vi "CSM - State Dashboard - DebugTool.vi"() -> ()   [LabVIEW 2014]
uses:
  _Support/Typedef/_CSM_GlobalLog_MSG.ctl
  _Support/Typedef/_CSM_GlobalLog_MSG_TYPE.ctl
  _Support/GlobalEvent/FGV-GlobalEventRef.vi
  <resource>/dialog/lvconfig.llb/LV Config Write Numeric (I32).vi
  <resource>/dialog/lvconfig.llb/LV Config Read Numeric (I32).vi
  _Support/jkism-tool-support.lvlib
  Communicable State Machine.lvlib
panel:
  in  "Clear JKISM":bool
  out "Dashboard":T1(array[cluster])
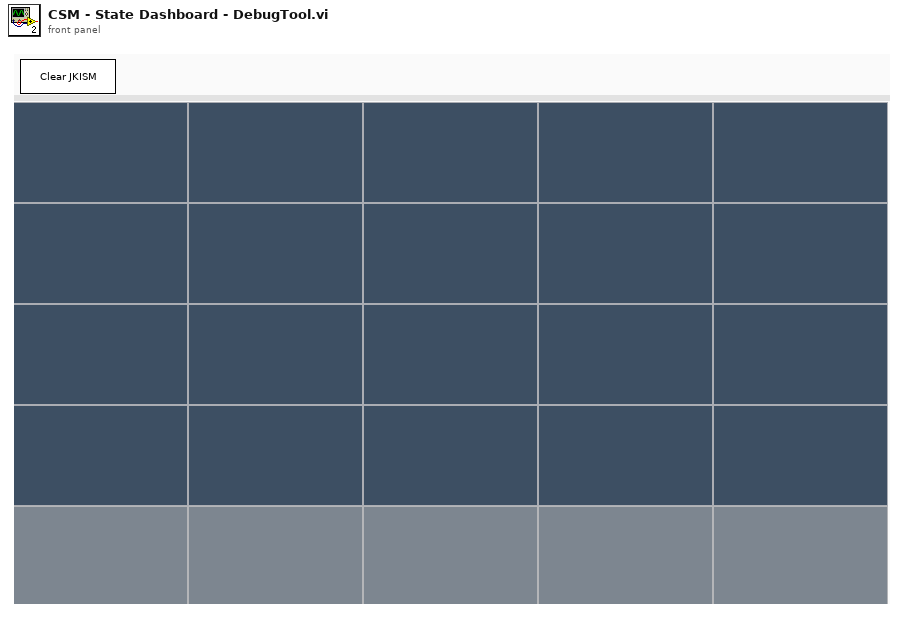
[diagram p1: front panel]
types:
  T1 = cluster{"Label":string, "Value":string, "String":string}[][]
  T2 = enum32{"Invalid", "Standard", "Closed", "Hidden", "Minimized", "Maximized"}
  T3 = enum32{"invalid app kind", "Development System", "Run Time System", "Student Edition", "Embedded LabVIEW", "Evaluation", "Custom"}
  T4 = typedef "Communicable State Machine.lvlib/_CSM_GlobalLog_MSG.ctl" = cluster{"Name(\"\" to use uuid)":string, "Current State":string, "Arguments":string, "Argument - State":string, "From Who":string, "Complete(T)/Start(F)":bool, "Type":T5}
  T5 = typedef "Communicable State Machine.lvlib/_CSM_GlobalLog_MSG_TYPE.ctl" = enum16{"User Log", "State Change", "Status", "Interrupt", "Register", "Unregister"}
  T6 = cluster{"Label":string, "Value":string, "String":string}
  T7 = typedef "JKI State Machine++.lvlib/_JKISM_GlobalLog_MSG_TYPE.ctl" = enum16{"User Log", "State Change", "Status", "Interrupt", "Register", "Unregister"}
  T8 = cluster{"Core":cluster{"Current VI Reference":refnum<vi>, "Close Panel on Exit?":bool}, "Global-DataTable":string[][], "NumCols":i16, "NumRows":i16, "JKISM Global Log Event":refnum<user-event>, "Log":T4}
  T9 = cluster{"Current VI Reference":refnum<vi>, "Close Panel on Exit?":bool}
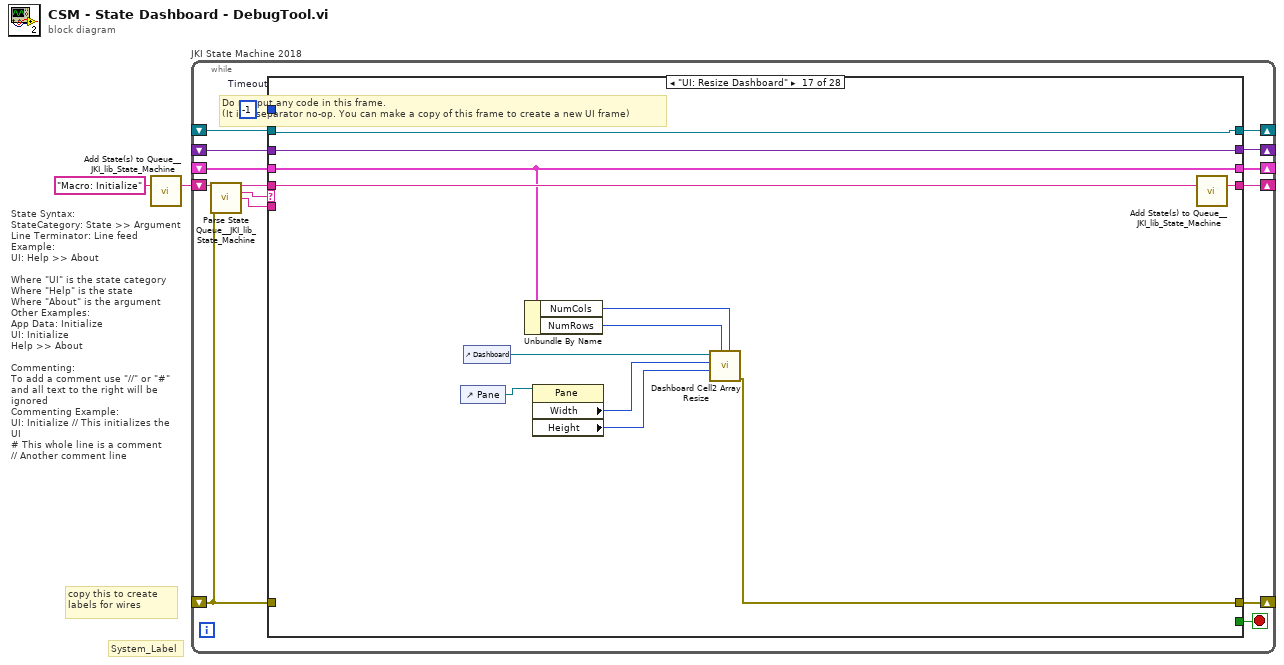
[diagram p0: block diagram]
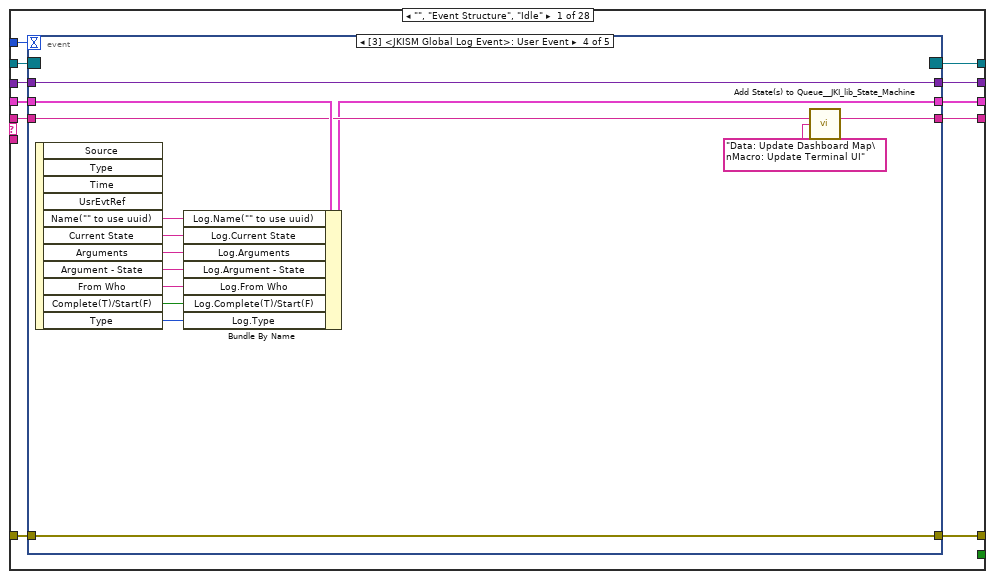
[diagram p2: hidden frame]
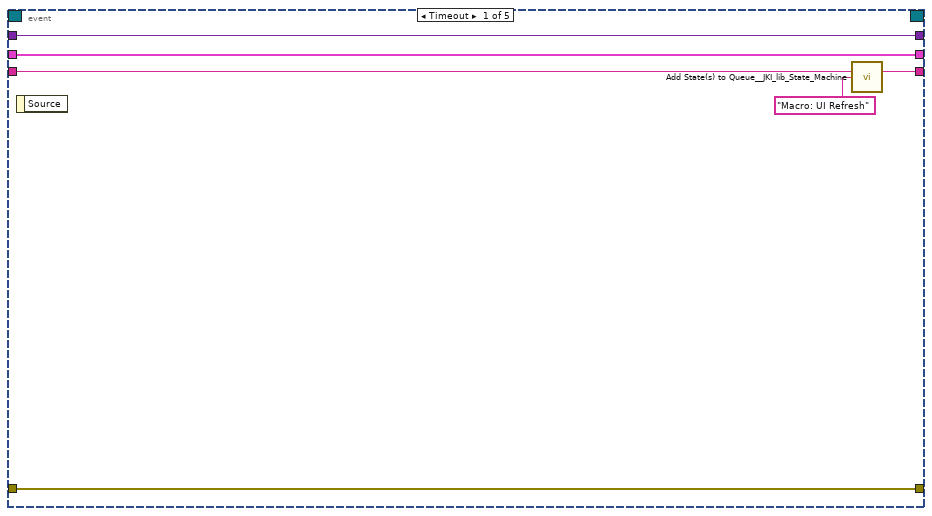
[diagram p3: hidden frame]
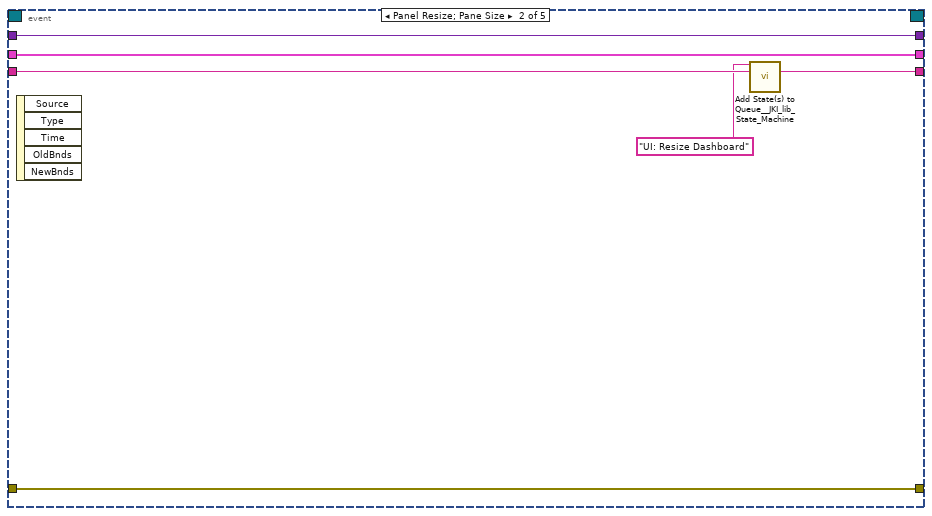
[diagram p4: hidden frame]
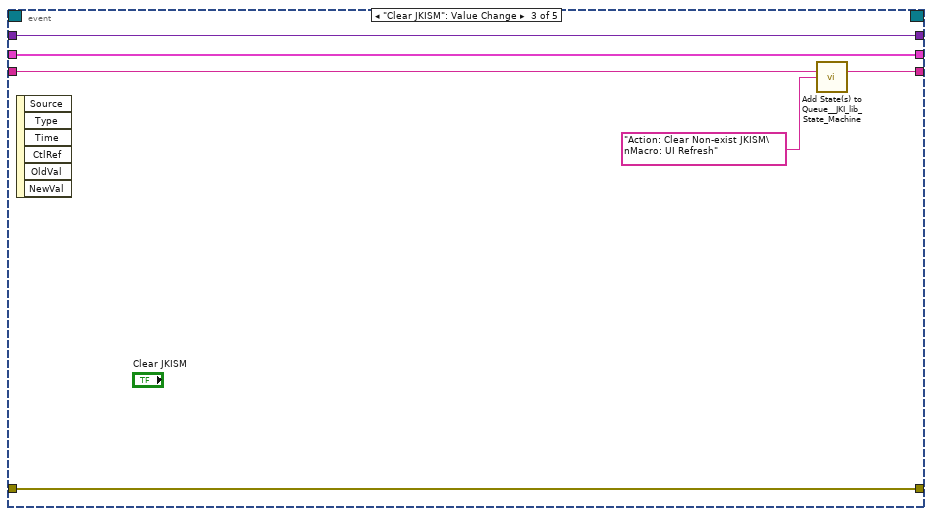
[diagram p5: hidden frame]
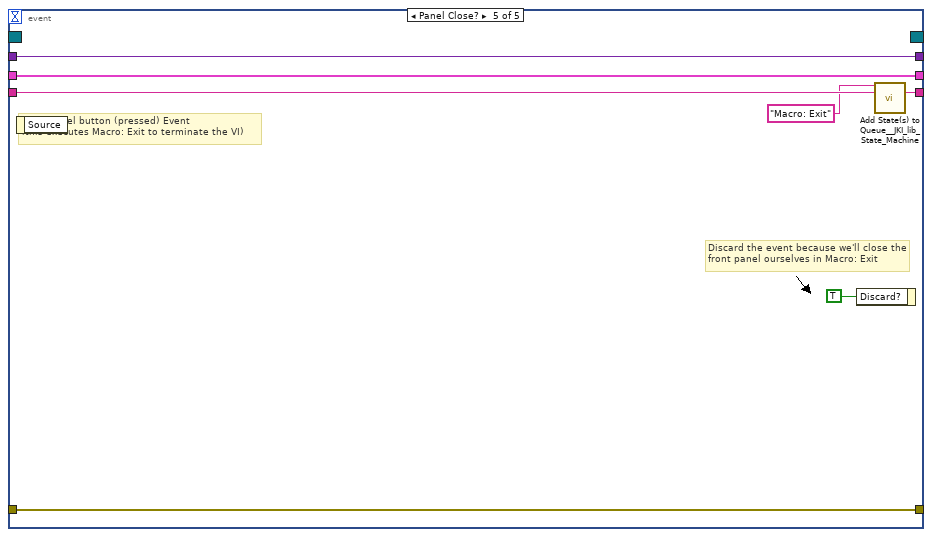
[diagram p6: hidden frame]
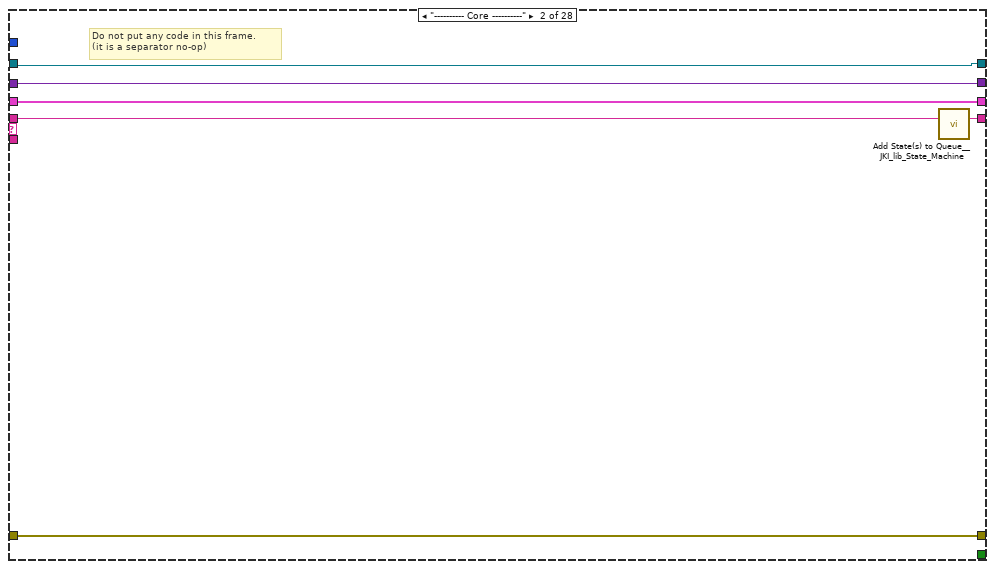
[diagram p7: hidden frame]
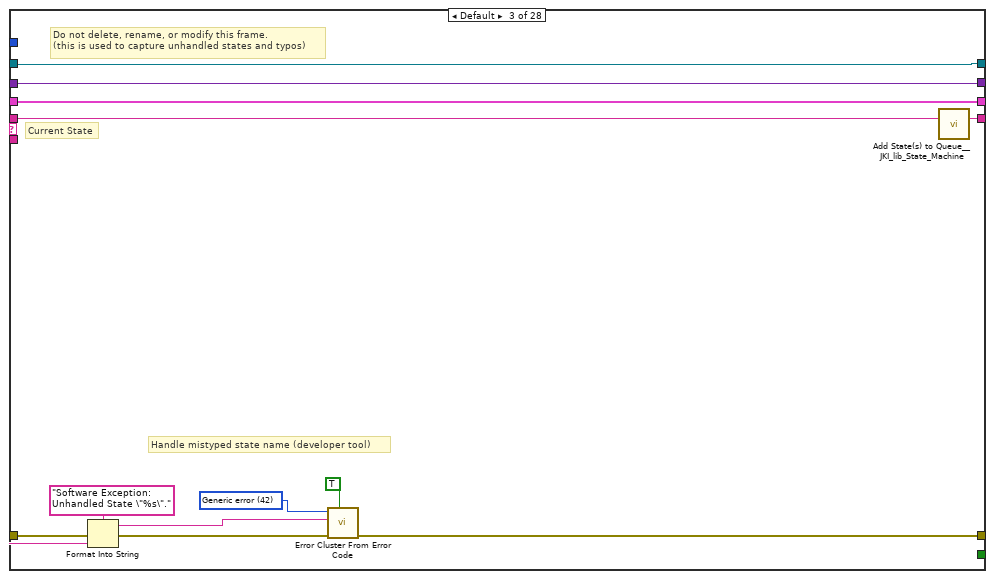
[diagram p8: hidden frame]
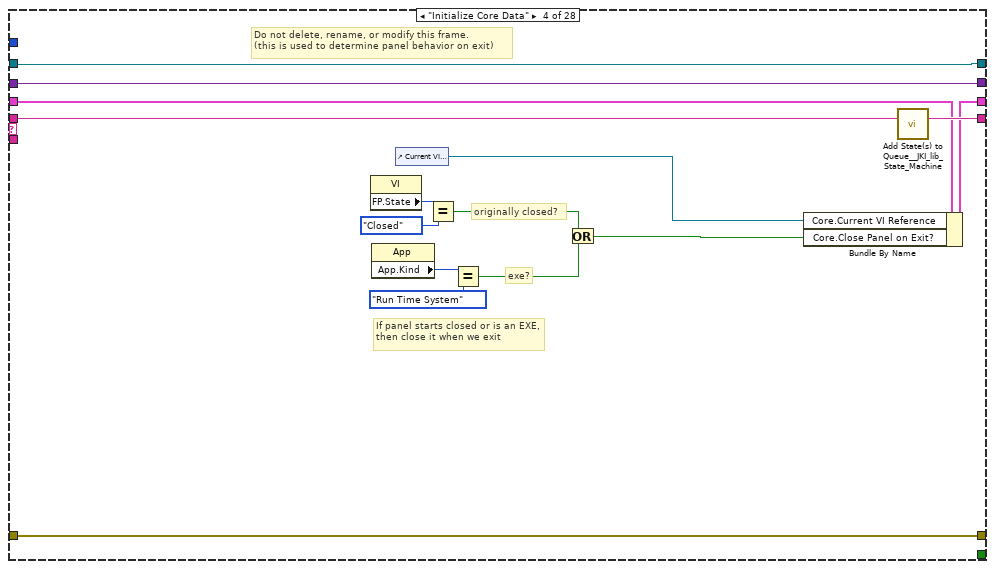
[diagram p9: hidden frame]
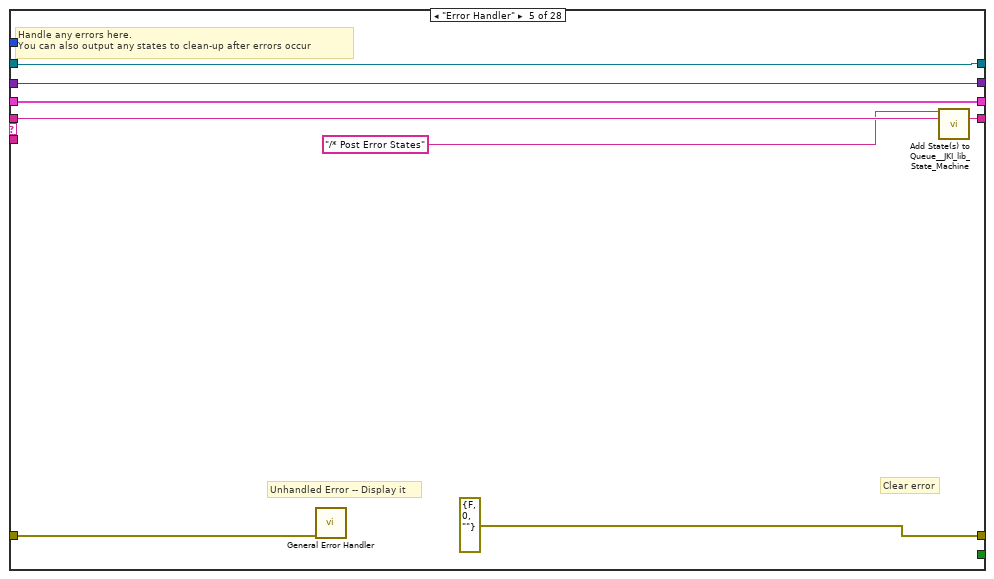
[diagram p10: hidden frame]
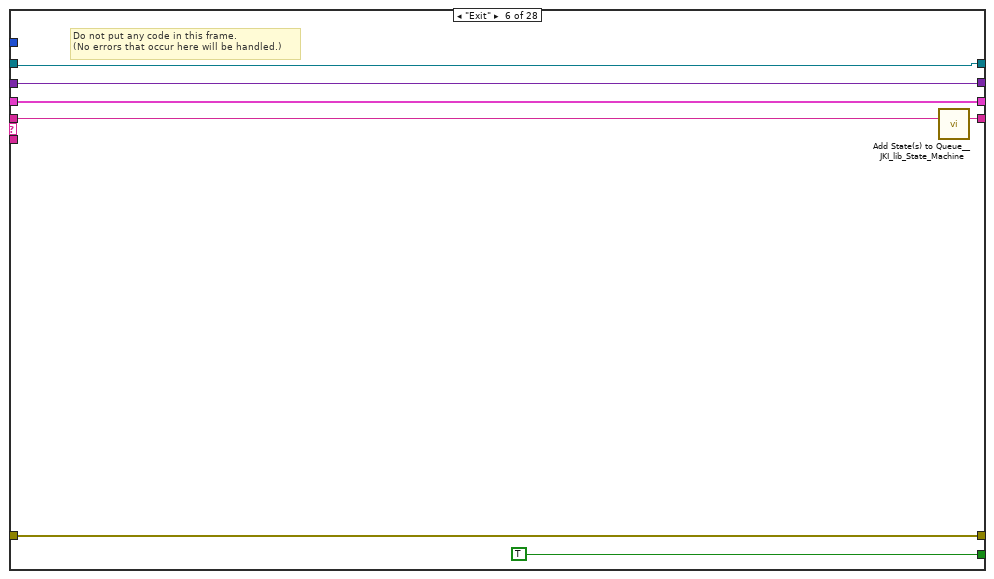
[diagram p11: hidden frame]
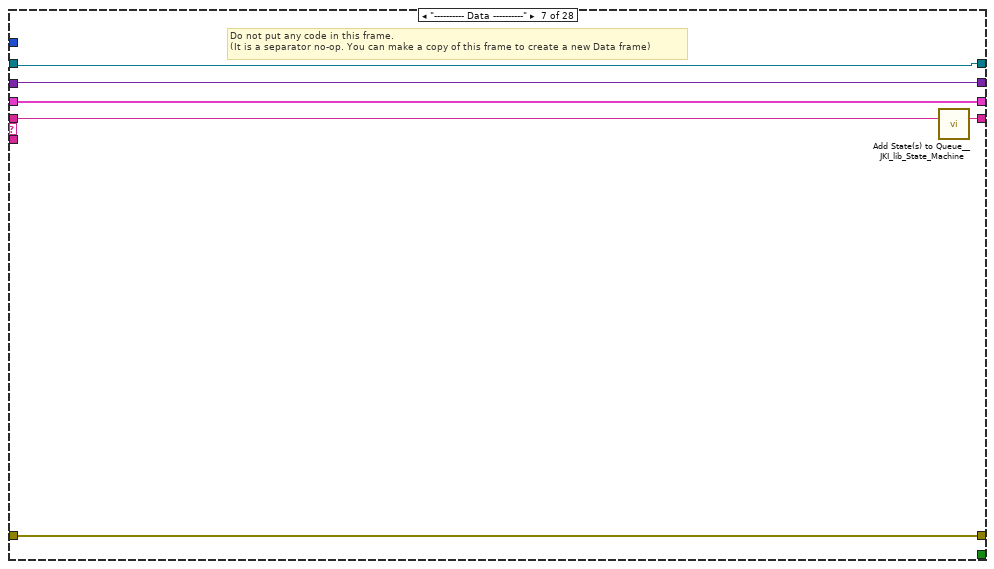
[diagram p12: hidden frame]
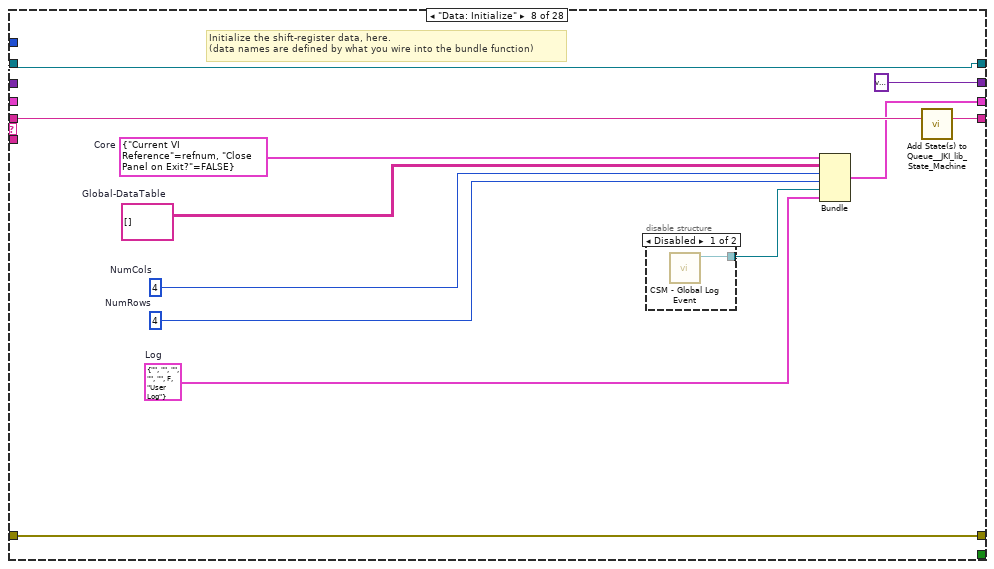
[diagram p13: hidden frame]
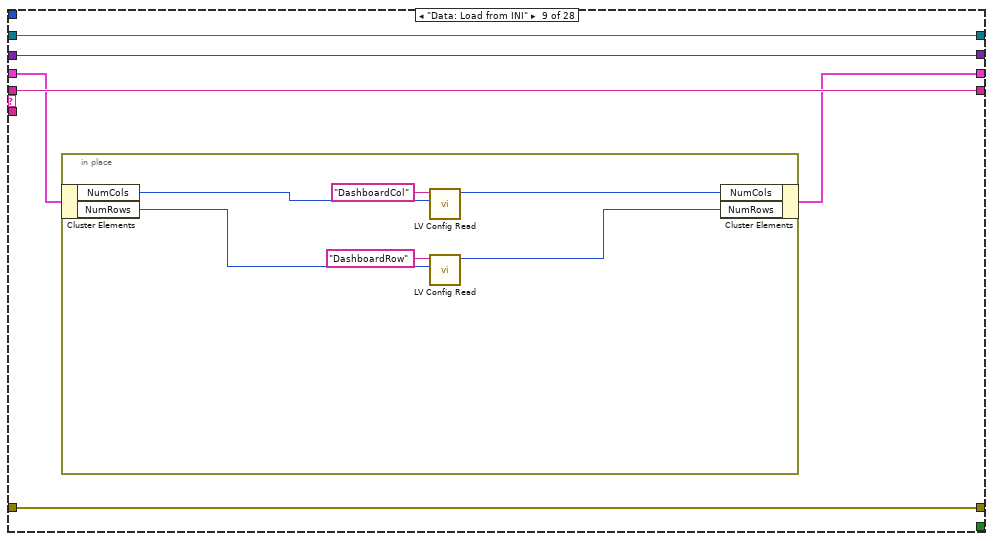
[diagram p15: hidden frame]
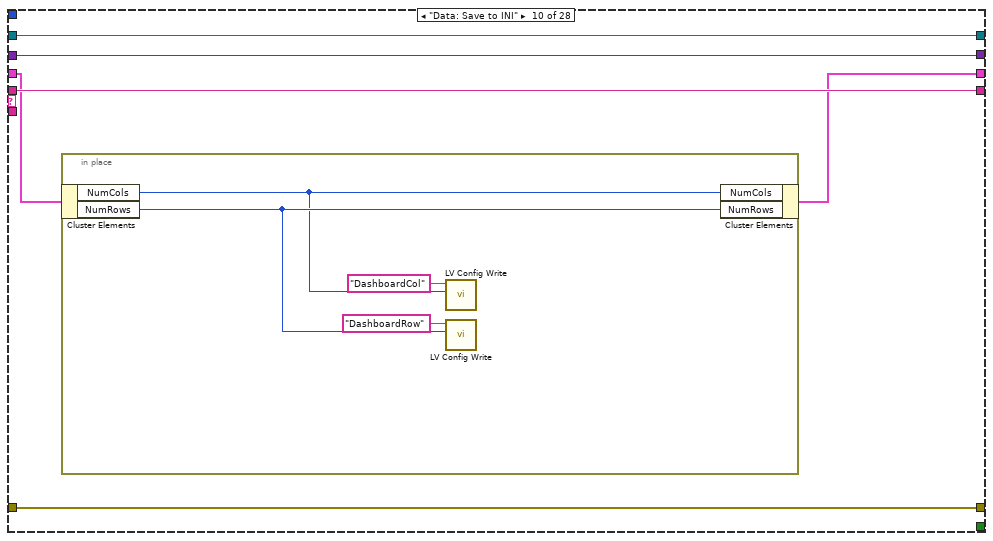
[diagram p16: hidden frame]
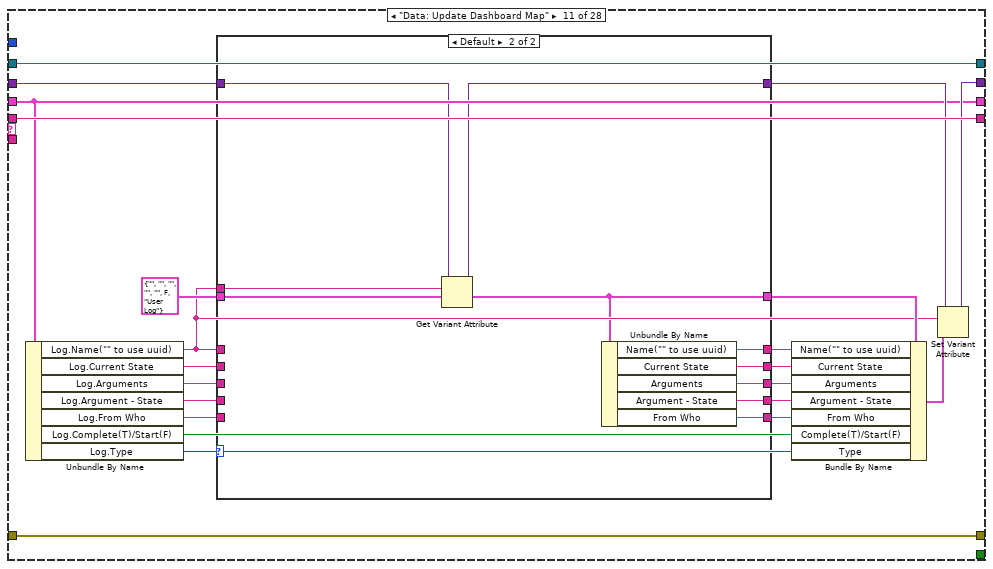
[diagram p17: hidden frame]
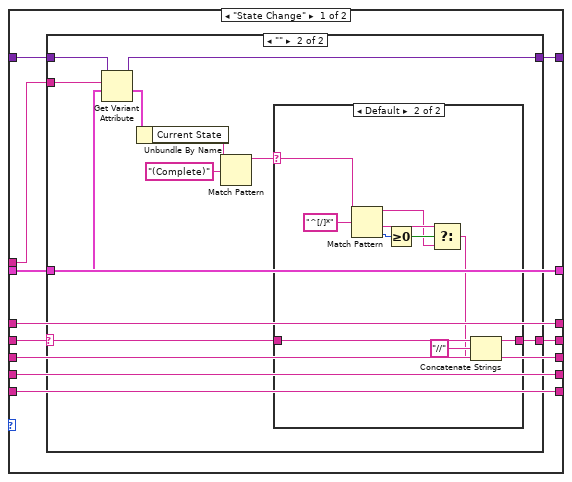
[diagram p18: hidden frame]
diagram:
  # "State Syntax:\nStateCategory: State >> Argument\nLine Terminator: Line feed\nExample:\nUI: Help >> About\n\nWhere \"UI\" is the state category\nWhere \"Help\" is the state\nWhere \"About\" is the argument\nOther Examples:\nApp Data: Initialize\nUI: Initialize\nHelp >> About\n\nCommenting:\nTo add a comment use \"//\" or \"#\" and all text to the right will be ignored\nCommenting Example:\nUI: Initialize // This initializes the UI\n# This whole line is a comment\n// Another comment line"
  # "copy this to create labels for wires"
  # "System_Label"
  n1 = call <vilib>:"Add State(s) to Queue__JKI_lib_State_Machine.vi"("State(s) in (\"\")"="Macro: Initialize") -> ("States Out"=w1:string)  [unwired: 14 in]
  n2 = while "JKI State Machine 2018" {
    shift-right: [w10] -> _
    shift-left: _ -> [w9]
    shift-right: [w13] -> _
    shift-left: _ -> [w7]
    shift-right: [w12] -> _
    shift-left: w1 -> [w14]
    shift-right: [w6] -> _
    shift-left: _ -> [w5]
    shift-right: [w4] -> _
    shift-left: _ -> [w3]
    stop <- w11 stop-if-true
    w8 = -1  # Timeout
    n3 = call <vilib>:"Parse State Queue__JKI_lib_State_Machine.vi"("State Queue"=w14, "Error In (no error)"=w7) -> ("Remaining States"=w16:string, "Current State"=w17:string, "Arguments"=w15:string)  [unwired: 11 in]
    n4 = case shown="\"UI: Resize Dashboard\"" w17 {
      selector: w17 -> [_ _ w76 _ _ _ _ _ _ _ _ _ _ _ _ _ _ _ _ _ _ _ _ _ _ _ _ _]
      tunnel: w16 -> [w28 w73 w80 w101 w109 w116 w122 w134 w140 w152 w178 w231 w237 w246 w258 w271 w348 w363 w373 w381 w389 w396 w403 w411 w418 w431 w435 w446]
      tunnel: w15 -> [_ _ _ _ _ _ _ _ _ _ _ _ _ _ w253 w265 _ _ _ _ _ _ _ _ _ _ _ _]
      tunnel: w9 -> [w26 w70 w78 w94 w106 w114 w119 _ w139 w151 w165 w226 w234 w242 w256 w267 w344 w360 w372 w380 w385 w393 w400 w406 w415 w428 w434 w445]
      tunnel: [w25 w71 w82 w98 errorcluster {"status"=FALSE, "code"=0, "source"=""} ("error out") w113 w120 w130 w141 w153 w179 w225 w235 w244 w254 w268 w345 w361 w374 w382 w390 w394 w401 w409 w416 w429 w436 w447] -> w13
      tunnel: w7 -> [w24 w71 w81 w98 w105 w113 w120 w130 w141 w153 w179 w228 w235 w244 w255 w269 _ w361 w374 w382 w390 w394 w401 w409 w416 w429 w436 w447]
      tunnel: [w27 w72 w79 w100 w108 w115 w121 w133 w140 w152 w178 w230 w236 w245 w257 w270 w347 w362 w373 w381 w389 w395 w402 w410 w417 w430 w435 w446] -> w12
      tunnel: [_ _ _ _ _ TRUE _ _ _ _ _ _ _ _ _ _ _ _ _ _ _ _ _ _ _ _ _ _] -> w11
      tunnel: [w23 w70 w78 w99 w106 w114 w119 w132 w138 w150 w165 w226 w234 w242 w256 w267 w344 w360 w372 w376 w385 w393 w400 w406 w415 w428 w434 w445] -> w10
      tunnel: w8 -> [w22 _ _ _ _ _ _ _ _ _ _ _ _ _ _ _ _ _ _ _ _ _ _ _ _ _ _ _]
      tunnel: [w20 w69 w75 w88 w103 w111 w118 variant w137 w149 w166 w224 w233 w239 w252 w264 w341 w355 w371 w379 w388 w392 w398 w405 w413 w421 w433 w441] -> w6
      tunnel: w5 -> [w21 w69 w75 w88 w103 w111 w118 _ w137 w149 w167 w224 w233 w239 w252 w264 w341 w354 w371 w379 w388 w392 w398 w405 w413 w421 w433 w443]
      tunnel: [w18 w68 w74 w87 w102 w110 w117 w125 w136 w148 w177 w223 w232 w238 w251 w263 w340 w351 w370 w377 w387 w391 w397 w404 w412 w420 w432 w444] -> w4
      tunnel: w3 -> [w19 w68 w74 w87 w102 w110 w117 w125 w136 w148 w177 w223 w232 w238 w251 w263 w340 w351 w370 _ w387 w391 w397 w404 w412 w420 w432 w444]
      frame "", "Event Structure", "Idle" {
        n5 = event shown="[3] <JKISM Global Log Event>: User Event" {
          selector: w19 -> [_ _ _ _ _]
          dyn-events: [_ _ _ _ _] -> w18
          timeout: w22 -> [_ _ _ _ _]
          tunnel: w28 -> [w34 w37 w43 w55 w67]
          tunnel: [w33 w38 w42 w59 w66] -> w27
          tunnel: w26 -> [w31 w39 w45 w56 w65]
          tunnel: [w32 w40 w46 w60 w62] -> w25
          tunnel: w24 -> [w32 w40 w46 w60 w62]
          tunnel: [w31 w39 w45 w54 w65] -> w23
          tunnel: w21 -> [w29 w35 w44 w57 w61]
          tunnel: [w29 w35 w44 w57 w61] -> w20
          event Timeout {
            n6 = event-data() -> ()  [unwired: 1 in, 1 out]
            n7 = call <vilib>:"Add State(s) to Queue__JKI_lib_State_Machine.vi"("State(s) in (\"\")"=w34, "State(s) at Back (\"\")"="Macro: UI Refresh" ("State(s) in Front (\"\")")) -> ("States Out"=w33:string)  [unwired: 13 in]
          }
          event Panel Resize; Pane Size {
            n8 = event-data() -> ()  [unwired: 1 in, 5 out]
            n9 = call <vilib>:"Add State(s) to Queue__JKI_lib_State_Machine.vi"("State(s) in Front (\"\")"="UI: Resize Dashboard" ("State(s) in Front (\"\")"), "State(s) in (\"\")"=w37) -> ("States Out"=w38:string)  [unwired: 13 in]
          }
          event "Clear JKISM": Value Change {
            n10 = event-data() -> ()  [unwired: 1 in, 6 out]
            n11 = call <vilib>:"Add State(s) to Queue__JKI_lib_State_Machine.vi"("State(s) in (\"\")"=w43, "State(s) at Back (\"\")"="Action: Clear Non-exist JKISM\nMacro: UI Refresh" ("State(s) at Back (\"\")")) -> ("States Out"=w42:string)  [unwired: 13 in]
          }
          event User Event {
            n12 = event-data() -> ("Name(\"\" to use uuid)"=w48:string, "Current State"=w49:string, "Arguments"=w50:string, "Argument - State"=w51:string, "From Who"=w52:string, "Complete(T)/Start(F)"=w53:bool, "Type"=w47:T7)  [unwired: 1 in, 4 out]
            n13 = Bundle By Name(cluster=w56, "Log.Name(\"\" to use uuid)"=w48, "Log.Current State"=w49, "Log.Arguments"=w50, "Log.Argument - State"=w51, "Log.From Who"=w52, "Log.Complete(T)/Start(F)"=w53, "Log.Type"=w47) -> (w54:T8)
            n14 = call <vilib>:"Add State(s) to Queue__JKI_lib_State_Machine.vi"("State(s) in (\"\")"=w55, "State(s) at Back (\"\")"="Data: Update Dashboard Map\nMacro: Update Terminal UI" ("State(s) at Back (\"\")")) -> ("States Out"=w59:string)  [unwired: 13 in]
          }
          event Panel Close? {
            # "Discard the event because we'll close the front panel ourselves in Macro: Exit"
            # "Close Panel button (pressed) Event\n(this executes Macro: Exit to terminate the VI)"
            n15 = event-data() -> ()  [unwired: 1 in, 1 out]
            n16 = event-data("Discard?"=TRUE) -> ()  [unwired: 1 in, 1 out]
            n17 = call <vilib>:"Add State(s) to Queue__JKI_lib_State_Machine.vi"("State(s) in Front (\"\")"="Macro: Exit", "State(s) in (\"\")"=w67) -> ("States Out"=w66:string)  [unwired: 13 in]
          }
        }
      }
      frame "---------- Core ----------" {
        # "Do not put any code in this frame.\n(it is a separator no-op)"
        n18 = call <vilib>:"Add State(s) to Queue__JKI_lib_State_Machine.vi"("State(s) in (\"\")"=w73) -> ("States Out"=w72:string)  [unwired: 14 in]
      }
      frame Default {
        w85 = 42 items=["No error", "Argument error", "Memory is full", "Out of zone", "End of file", "File already open", "Generic file I/O error", "File not found", "File permission error", "Disk is full", "Duplicate path", "Too many files open", "System feature not enabled", "Resource file not found", "Cannot add resource", "Resource not found", "Image not found", "Image memory error", "Pen does not exist", "Config type invalid", "Config token not found", "Config parse error", "Config memory error", "Bad external code format", "Bad external code offset", "External code not present", "Null window", "Destroy window error", "Null menu", "Print aborted", "Bad print record", "Print driver error", "Windows error during printing", "Memory error during printing", "Print dialog error", "Generic print error", "Invalid device refnum", "Device not found", "Device parameter error", "Device unit error", "Cannot open device", "Device call aborted", "Generic error", "Cancelled by user", "Object ID too low", "Object ID too high", "Object not in heap", "Unknown heap", "Unknown object (invalid DefProc)", "Unknown object (DefProc not in table)", "Message out of range", "Invalid (null) method", "Unknown message", "Manager call not supported", "Bad address", "Network operation in progress", "Network operation timed out", "Connection is busy", "Network attribute not supported", "Network error", "Address in use", "System out of memory", "Connection aborted", "Connection refused", "Not connected", "Already connected", "Connection closed", "Initialization error (interapplication manager)", "Bad occurrence", "Wait on unbound occurrence handler", "Occurrence queue overflow", "Datalog type conflict", "Unused", "Unrecognized type (interapplication manager)", "Memory corrupt", "Failed to make temporary DLL", "Old CIN version", "Drag socket not found", "Failed to load drop-object", "Failed to register OLE object", "Failed to release OLE object", "Format specifier type mismatch", "Unknown format specifier", "Too few format specifiers", "Too many format specifiers", "Scan failed", "Newer CIN version", "Error converting to variant", "Runtime menu error", "Password tampered", "Variant attribute not found", "Incompatible variant data type", "Event data is not available", "Event Store is not present", "Occurrence is not found", "Event Queue is not created", "Event info is not available", "Refnum passed is NULL", "Error retrieving Class GUID", "Error retrieving CoClass GUID", "Error retrieving TypeLib GUID.", "Bad built application magic bytes.", "Specific driver is different from the specific driver associated with the Logical Name.", "There is no session opened to the class driver.", "Max Error", "MAX - Error with config objects", "MAX - Error loading configuration", "MAX - Group not supported"]
        # "Current State"
        # "Do not delete, rename, or modify this frame.\n(this is used to capture unhandled states and typos)"
        # "Handle mistyped state name (developer tool)"
        n19 = Format Into String(format string="Software Exception: Unhandled State \"%s\"." ("message"), error in=w81, w76) -> (resulting string=w84:string, error out=w83:errorcluster)  [unwired: 1 in]
        n20 = call <vilib>:"Error Cluster From Error Code.vi"("show call chain? (False)"=TRUE, "error in (no error)"=w83, "error message (\"\")"=w84, "error code (0)"=w85) -> ("error out"=w82:errorcluster)  [unwired: 5 in]
        n21 = call <vilib>:"Add State(s) to Queue__JKI_lib_State_Machine.vi"("State(s) in (\"\")"=w80) -> ("States Out"=w79:string)  [unwired: 14 in]
      }
      frame "Initialize Core Data" {
        # "Do not delete, rename, or modify this frame.\n(this is used to determine panel behavior on exit)"
        # "originally closed?"
        # "exe?"
        # "If panel starts closed or is an EXE, then close it when we exit"
        n22 = property class="VI"() -> ("FP.State"=w91:T2)  [unwired: 2 in, 2 out]
        n23 = property class="App"() -> ("App.Kind"=w97:T3)  [unwired: 2 in, 2 out]
        n24 = control-ref of="Current VI Reference"() -> (w92:refnum<vi>)
        n25 = Equal?(x=w91, y=T2."Closed" ("Front Panel Window:State")) -> (x = y?=w89:bool)
        n26 = Equal?(x=w97, y=T3."Run Time System" ("Application:Kind")) -> (x = y?=w95:bool)
        n27 = Or(x=w89, y=w95) -> (x .or. y?=w93:bool)
        n28 = Bundle By Name(cluster=w94, "Core.Current VI Reference"=w92, "Core.Close Panel on Exit?"=w93) -> (w99:T8)
        n29 = call <vilib>:"Add State(s) to Queue__JKI_lib_State_Machine.vi"("State(s) in (\"\")"=w101) -> ("States Out"=w100:string)  [unwired: 14 in]
      }
      frame "Error Handler" {
        # "Unhandled Error -- Display it"
        # "Handle any errors here.\nYou can also output any states to clean-up after errors occur"
        # "Clear error"
        n30 = call <vilib>:"General Error Handler.vi"("error in (no error)"=w105) -> ()  [unwired: 10 in, 5 out]
        n31 = call <vilib>:"Add State(s) to Queue__JKI_lib_State_Machine.vi"("State(s) in Front (\"\")"="/* Post Error States", "State(s) in (\"\")"=w109) -> ("States Out"=w108:string)  [unwired: 13 in]
      }
      frame "Exit" {
        # "Do not put any code in this frame.\n(No errors that occur here will be handled.)"
        n32 = call <vilib>:"Add State(s) to Queue__JKI_lib_State_Machine.vi"("State(s) in (\"\")"=w116) -> ("States Out"=w115:string)  [unwired: 14 in]
      }
      frame "---------- Data ----------" {
        # "Do not put any code in this frame.\n(It is a separator no-op. You can make a copy of this frame to create a new Data frame)"
        n33 = call <vilib>:"Add State(s) to Queue__JKI_lib_State_Machine.vi"("State(s) in (\"\")"=w122) -> ("States Out"=w121:string)  [unwired: 14 in]
      }
      frame "Data: Initialize" {
        w123 = T4 {"Name(\"\" to use uuid)"="", "Current State"="", "Arguments"="", "Argument - State"="", "From Who"="", "Complete(T)/Start(F)"=FALSE, "Type"=enum."User Log"}  # Log
        w128 = i16 4  # NumCols
        w127 = i16 4  # NumRows
        w129 = string[][] []  # Global-DataTable
        w131 = T9 {"Current VI Reference"=refnum, "Close Panel on Exit?"=FALSE}  # Core
        # "Initialize the shift-register data, here.\n(data names are defined by what you wire into the bundle function)"
        n34 = disable-structure shown="Disabled" {
          disable-tunnel: [w135 _] -> w124
          frame Disabled {
            n35 = call "CSM - Global Log Event.vi"() -> ("JKISM Global Log Event"=w135:refnum<user-event>)  [unwired: 10 in, 1 out]
          }
          frame Enabled {
          }
        }
        n36 = Bundle("Core"=w131, "Global-DataTable"=w129, "NumCols"=w128, "NumRows"=w127, "JKISM Global Log Event"=w124, "Log"=w123) -> (w132:T8)  [unwired: 1 in]
        n37 = call <vilib>:"Add State(s) to Queue__JKI_lib_State_Machine.vi"("State(s) in (\"\")"=w134) -> ("States Out"=w133:string)  [unwired: 14 in]
      }
      frame "Data: Load from INI" {
        n38 = in-place {
          n39 = in-place-cluster #1(w139) -> ("NumCols"=w143:i16, "NumRows"=w146:i16)
          n40 = call-poly <resource>:"LV Config Read.vi"("default value"=w143, "key"="DashboardCol") -> ("value"=w142:i32)  [unwired: 3 in, 2 out]
          n41 = call-poly <resource>:"LV Config Read.vi"("default value"=w146, "key"="DashboardRow") -> ("value"=w145:i32)  [unwired: 3 in, 2 out]
          n42 = in-place-cluster #1("NumCols"=w142, "NumRows"=w145) -> (w138:T8)
        }
      }
      frame "Data: Save to INI" {
        n43 = in-place {
          n44 = in-place-cluster #2(w151) -> ("NumCols"=w154:i16, "NumRows"=w155:i16)
          n45 = call-poly <resource>:"LV Config Write.vi"("value"=w154, "key"="DashboardCol") -> ()  [unwired: 5 in, 1 out]
          n46 = call-poly <resource>:"LV Config Write.vi"("value"=w155, "key"="DashboardRow") -> ()  [unwired: 5 in, 1 out]
          n47 = in-place-cluster #2("NumCols"=w154, "NumRows"=w155) -> (w150:T8)
        }
      }
      frame "Data: Update Dashboard Map" {
        n48 = Unbundle By Name(w165) -> ("Log.Name(\"\" to use uuid)"=w160:string, "Log.Current State"=w164:string, "Log.Arguments"=w163:string, "Log.Argument - State"=w162:string, "Log.From Who"=w161:string, "Log.Complete(T)/Start(F)"=w158:bool, "Log.Type"=w159:T5)
        n49 = case shown="Default" w159 {
          tunnel: w167 -> [w185 w222]
          tunnel: [w184 w221] -> w175
          tunnel: T4 {"Name(\"\" to use uuid)"="", "Current State"="", "Arguments"="", "Argument - State"="", "From Who"="", "Complete(T)/Start(F)"=FALSE, "Type"=enum."User Log"} ("Cross JKI State Machine Data") -> [w182 w220]
          tunnel: w160 -> [w183 w219]
          tunnel: w161 -> [w189 _]
          tunnel: [w189 w218] -> w173
          tunnel: w162 -> [w188 _]
          tunnel: [w188 w217] -> w172
          tunnel: w163 -> [w187 _]
          tunnel: [w187 w216] -> w171
          tunnel: w164 -> [w181 _]
          tunnel: [w180 w213] -> w170
          tunnel: w160 -> [w186 _]
          tunnel: [w186 w214] -> w169
          tunnel: [w182 w215] -> w168
          frame "State Change" {
            n50 = case shown="\"\"" w181 {
              selector: w181 -> [w190 w193]
              tunnel: w185 -> [w191 w201]
              tunnel: [w191 w200] -> w184
              tunnel: w183 -> [_ w199]
              tunnel: w182 -> [_ w197]
              tunnel: [w190 w192] -> w180
              frame Default {
              }
              frame "" {
                n51 = Get Variant Attribute(Variant=w201, name=w199, default value (empty Variant)=w197) -> (duplicate Variant=w200:variant, value=w198:T4)  [unwired: 1 in, 2 out]
                n52 = Unbundle By Name(w198) -> ("Current State"=w196:string)
                n53 = Match Pattern(string=w196, regular expression="(Complete)") -> (before substring=w194:string)  [unwired: 1 in, 3 out]
                n54 = case shown="Default" w194 {
                  selector: w194 -> [_ w208]
                  tunnel: w193 -> [w202 w212]
                  tunnel: [w202 w211] -> w192
                  frame "" {
                  }
                  frame Default {
                    n55 = Match Pattern(string=w208, regular expression="^[/]*") -> (before substring=w203:string, after substring=w205:string, offset past match=w207:i32)  [unwired: 1 in, 1 out]
                    n56 = Greater Or Equal To 0?(x=w207) -> (x >= 0?=w206:bool)
                    n57 = Select(t=w205, s=w206, f=w203) -> (s? t:f=w204:string)
                    n58 = Concatenate Strings(w212, "//" ("string"), w204) -> (w211:string)
                  }
                }
              }
            }
          }
          frame Default {
            n59 = Get Variant Attribute(Variant=w222, name=w219, default value (empty Variant)=w220) -> (duplicate Variant=w221:variant, value=w215:T4)  [unwired: 1 in, 2 out]
            n60 = Unbundle By Name(w215) -> ("Name(\"\" to use uuid)"=w214:string, "Current State"=w213:string, "Arguments"=w216:string, "Argument - State"=w217:string, "From Who"=w218:string)
          }
        }
        n61 = Bundle By Name(cluster=w168, "Name(\"\" to use uuid)"=w169, "Current State"=w170, "Arguments"=w171, "Argument - State"=w172, "From Who"=w173, "Complete(T)/Start(F)"=w158, "Type"=w159) -> (w176:T4)
        n62 = Set Variant Attribute(Variant=w175, name=w160, value=w176) -> (Variant out=w166:variant)  [unwired: 1 in, 2 out]
      }
      frame "Data: Cleanup" {
        # "Cleanup any data and references, here.\n(this is called automatically, by the Macro: Exit)"
        n63 = Unbundle By Name(w226) -> ("Core.Current VI Reference"=w229:refnum<vi>)
        n64 = Close Reference(reference=w229, error in (no error)=w228) -> (error out=w227:errorcluster)
        n65 = Merge Errors(w227) -> (w225:errorcluster)
        n66 = call <vilib>:"Add State(s) to Queue__JKI_lib_State_Machine.vi"("State(s) in (\"\")"=w231) -> ("States Out"=w230:string)  [unwired: 14 in]
      }
      frame "---------- UI ----------" {
        # "Do not put any code in this frame.\n(It is a separator no-op. You can make a copy of this frame to create a new UI frame)"
        n67 = call <vilib>:"Add State(s) to Queue__JKI_lib_State_Machine.vi"("State(s) in (\"\")"=w237) -> ("States Out"=w236:string)  [unwired: 14 in]
      }
      frame "UI: Initialize" {
        # "Initialize the User Interface, here.\n(this is called automatically, by the Macro: Init)"
        n68 = invoke class="VI" method="Default Vals.Reinit All"() -> (error out=w243:errorcluster)  [unwired: 3 in, 2 out]
        n69 = Unbundle By Name(w242) -> ("NumRows"=w241:i16, "NumCols"=w240:i16)
        n70 = flat-sequence {
          tunnel: w243 -> [_]
          tunnel: w241 -> [w248]
          tunnel: w240 -> [w247]
          frame #0 {
            n71 = Initialize Array(T6 {"Label"="", "Value"="", "String"=""} ("Dashboard"), w248, w247) -> (w249:T1)
            n72 = local write "Dashboard"(w249) -> ()
          }
        }
        n73 = call <vilib>:"Add State(s) to Queue__JKI_lib_State_Machine.vi"("State(s) in (\"\")"=w246) -> ("States Out"=w245:string)  [unwired: 14 in]
      }
      frame "UI: Cursor Set" {
        # "Argument"
        # "Set and Unset Cursor Busy.\n(Usage: \"UI: Cursor Set >> Busy|Idle\")"
        n74 = case shown="\"Idle\", Default" w253 {
          tunnel: w255 -> [w260 w262]
          tunnel: [w259 w261] -> w254
          frame "Idle", Default {
            n75 = call <vilib>:"Unset Busy.vi"("error in (no error)"=w260) -> ("error out"=w259:errorcluster)  [unwired: 10 in]
          }
          frame "Busy" {
            n76 = call <vilib>:"Set Busy.vi"("error in (no error)"=w262) -> ("error out"=w261:errorcluster)  [unwired: 9 in, 1 out]
          }
        }
        n77 = call <vilib>:"Add State(s) to Queue__JKI_lib_State_Machine.vi"("State(s) in (\"\")"=w258) -> ("States Out"=w257:string)  [unwired: 14 in]
      }
      frame "UI: Front Panel State" {
        # "Argument"
        # "Set Front Panel Open or Closed\n(Usage: \"UI: Front Panel State >> Open|Close\")"
        n78 = Unbundle By Name(w267) -> ("Core.Current VI Reference"=w266:refnum<vi>)
        n79 = case shown="\"Minimize\", \"Minimized\"" w265 {
          tunnel: w269 -> [w277 w292 w303 w316 w329]
          tunnel: [w279 w293 w305 w318 w331] -> w268
          tunnel: w266 -> [w278 w290 w304 w317 w330]
          frame "Open", "Standard", Default {
            w272 = T2."Standard" ("State")
            n80 = property class="VI"(reference=w278, error in=w277) -> (reference out=w275:refnum<vi>, error out=w276:errorcluster, "FP.State"=w274:T2)
            n81 = Not Equal?(x=w274, y=w272) -> (x != y?=w273:bool)
            n82 = case shown="True" w273 {
              tunnel: [w283 w285] -> w279
              tunnel: w276 -> [w282 w285]
              tunnel: w275 -> [w281 _]
              tunnel: w272 -> [w280 _]
              frame True {
                n83 = invoke class="VI" method="FP.Open"(reference=w281, error in=w282, "Activate"=TRUE, "State"=w280) -> (error out=w283:errorcluster)  [unwired: 1 in, 4 out]
              }
              frame False {
              }
            }
          }
          frame "Close", "Closed" {
            n84 = property class="VI"(reference=w290, error in=w292) -> (reference out=w289:refnum<vi>, error out=w291:errorcluster, "FP.State"=w287:T2)
            n85 = Not Equal?(x=w287, y=T2."Closed" ("Front Panel Window:State")) -> (x != y?=w286:bool)
            n86 = case shown="True" w286 {
              tunnel: [w294 w297] -> w293
              tunnel: w291 -> [w294 w296]
              tunnel: w289 -> [_ w295]
              frame False {
              }
              frame True {
                n87 = invoke class="VI" method="FP.Close"(reference=w295, error in=w296) -> (error out=w297:errorcluster)  [unwired: 1 in, 2 out]
              }
            }
          }
          frame "Hidden", "Hide" {
            w298 = T2."Hidden" ("State")
            n88 = property class="VI"(reference=w304, error in=w303) -> (reference out=w301:refnum<vi>, error out=w302:errorcluster, "FP.State"=w300:T2)
            n89 = Not Equal?(x=w300, y=w298) -> (x != y?=w299:bool)
            n90 = case shown="True" w299 {
              tunnel: [w309 w310] -> w305
              tunnel: w302 -> [w308 w310]
              tunnel: w301 -> [w307 _]
              tunnel: w298 -> [w306 _]
              frame True {
                n91 = invoke class="VI" method="FP.Open"(reference=w307, error in=w308, "State"=w306) -> (error out=w309:errorcluster)  [unwired: 2 in, 4 out]
              }
              frame False {
              }
            }
          }
          frame "Minimize", "Minimized" {
            w311 = T2."Minimized" ("State")
            n92 = property class="VI"(reference=w317, error in=w316) -> (reference out=w314:refnum<vi>, error out=w315:errorcluster, "FP.State"=w313:T2)
            n93 = Not Equal?(x=w313, y=w311) -> (x != y?=w312:bool)
            n94 = case shown="True" w312 {
              tunnel: [w322 w323] -> w318
              tunnel: w315 -> [w321 w323]
              tunnel: w314 -> [w320 _]
              tunnel: w311 -> [w319 _]
              frame True {
                n95 = invoke class="VI" method="FP.Open"(reference=w320, error in=w321, "State"=w319) -> (error out=w322:errorcluster)  [unwired: 2 in, 4 out]
              }
              frame False {
              }
            }
          }
          frame "Maximize", "Maximized" {
            w324 = T2."Maximized" ("State")
            n96 = property class="VI"(reference=w330, error in=w329) -> (reference out=w327:refnum<vi>, error out=w328:errorcluster, "FP.State"=w326:T2)
            n97 = Not Equal?(x=w326, y=w324) -> (x != y?=w325:bool)
            n98 = case shown="True" w325 {
              tunnel: [w335 w336] -> w331
              tunnel: w328 -> [w334 w336]
              tunnel: w327 -> [w333 _]
              tunnel: w324 -> [w332 _]
              frame True {
                n99 = invoke class="VI" method="FP.Open"(reference=w333, error in=w334, "State"=w332) -> (error out=w335:errorcluster)  [unwired: 2 in, 4 out]
              }
              frame False {
              }
            }
          }
        }
        n100 = call <vilib>:"Add State(s) to Queue__JKI_lib_State_Machine.vi"("State(s) in (\"\")"=w271) -> ("States Out"=w270:string)  [unwired: 14 in]
      }
      frame "UI: Resize Dashboard" {
        # "Do not put any code in this frame.\n(It is a separator no-op. You can make a copy of this frame to create a new UI frame)"
        n101 = control-ref of="Pane"() -> (w337:refnum<vi>)
        n102 = control-ref of="Dashboard"() -> (w346:refnum<vi>)
        n103 = Unbundle By Name(w344) -> ("NumCols"=w342:i16, "NumRows"=w343:i16)
        n104 = property class="Pane"(reference=w337) -> ("Width"=w339:u32, "Height"=w338:u32)  [unwired: 1 in, 2 out]
        n105 = call "Dashboard Cell2 Array Resize.vi"("Num Columns"=w342, "Num Rows"=w343, "area height"=w338, "area width"=w339, "Array 2"=w346) -> ("error out"=w345:errorcluster)  [unwired: 6 in]
        n106 = call <vilib>:"Add State(s) to Queue__JKI_lib_State_Machine.vi"("State(s) in (\"\")"=w348) -> ("States Out"=w347:string)  [unwired: 14 in]
      }
      frame "UI: Update Dashboard" {
        # "Do not put any code in this frame.\n(It is a separator no-op. You can make a copy of this frame to create a new UI frame)"
        n107 = Get Variant Attribute(Variant=w354) -> (duplicate Variant=w355:variant, names=w353:string[], values=w352:variant[])  [unwired: 3 in, 1 out]
        n108 = Variant To Data(type=T4[] [], Variant=w352) -> (data=w349:T4[])  [unwired: 1 in, 1 out]
        n109 = for {
          tunnel: w353 -> [w368] mode=indexing
          tunnel: [w367] -> w359 mode=indexing
          tunnel: w349 -> [w366] mode=indexing
          n110 = Unbundle By Name(w366) -> ("Current State"=w365:string, "Arguments"=w364:string)  [unwired: 1 out]
          n111 = Bundle By Name(cluster=T6 {"Label"="", "Value"="", "String"=""}, "Label"=w368, "Value"=w365, "String"=w364) -> (w367:T6)
        }
        n112 = Unbundle By Name(w360) -> ("NumRows"=w357:i16, "NumCols"=w356:i16)
        n113 = Reshape Array(w359, w357, w356) -> (→"Dashboard":T1)
        n114 = call <vilib>:"Add State(s) to Queue__JKI_lib_State_Machine.vi"("State(s) in (\"\")"=w363) -> ("States Out"=w362:string)  [unwired: 14 in]
      }
      frame "--------- Event ---------" {
      }
      frame "Register User Event" {
        n115 = call "CSM - Global Log Event.vi"() -> ("Error out"=w378:errorcluster, "JKISM Global Log Event"=w375:refnum<user-event>)  [unwired: 10 in]
        n116 = register-events(error in=w378, w375) -> (reference out=w377:refnum<event-registration>)  [unwired: 1 in, 1 out]
        n117 = Bundle By Name(cluster=w380, "JKISM Global Log Event"=w375) -> (w376:T8)
      }
      frame "UnRegister User Event" {
        n118 = Unregister For Events(event registration refnum=w387) -> (error out=w386:errorcluster)  [unwired: 1 in]
        n119 = Unbundle By Name(w385) -> ("JKISM Global Log Event"=w384:refnum<user-event>)
        n120 = call "CSM - Destroy Global Log Event.vi"("Error in"=w386, "JKISM Global Log Event"=w384) -> ("Error out"=w383:errorcluster)  [unwired: 9 in]
        n121 = call <vilib>:"Clear Errors.vi"("error in (no error)"=w383) -> ()  [unwired: 5 in, 2 out]
      }
      frame "---------- Macro ----------" {
        # "Do not put any code in this frame.\n(It is a separator no-op. You can make a copy of this frame to create a new Macro frame)"
        n122 = call <vilib>:"Add State(s) to Queue__JKI_lib_State_Machine.vi"("State(s) in (\"\")"=w396) -> ("States Out"=w395:string)  [unwired: 14 in]
      }
      frame "Macro: Initialize" {
        # "Initialization Macro\n(This is called once, when the VI starts)"
        n123 = call <vilib>:"Add State(s) to Queue__JKI_lib_State_Machine.vi"("State(s) in Front (\"\")"="Data: Initialize\nInitialize Core Data\nData: Load from INI\nUI: Initialize\nUI: Resize Dashboard\nRegister User Event\n//UI: Front Panel State >> Open", "State(s) in (\"\")"=w403) -> ("States Out"=w402:string)  [unwired: 13 in]
      }
      frame "Macro: UI Refresh" {
        # "Do not put any code in this frame.\n(It is a separator no-op. You can make a copy of this frame to create a new Macro frame)"
        n124 = call <vilib>:"Add State(s) to Queue__JKI_lib_State_Machine.vi"("State(s) at Back (\"\")"="Macro: Update Terminal UI" ("State(s) in Front (\"\")")) -> ("States Out"=w408:string)  [unwired: 14 in]
        n125 = call <vilib>:"Add State(s) to Queue__JKI_lib_State_Machine.vi"("State(s) in Front (\"\")"=w408, "State(s) in (\"\")"=w411) -> ("States Out"=w410:string)  [unwired: 13 in]
      }
      frame "Macro: Update Terminal UI" {
        # "Do not put any code in this frame.\n(It is a separator no-op. You can make a copy of this frame to create a new Macro frame)"
        n126 = call <vilib>:"Add State(s) to Queue__JKI_lib_State_Machine.vi"("State(s) in Front (\"\")"="UI: Update Dashboard" ("State(s) in Front (\"\")"), "State(s) in (\"\")"=w418) -> ("States Out"=w417:string)  [unwired: 13 in]
      }
      frame "Macro: Exit" {
        # "Exit Macro\n(This is called once, when the VI exits)"
        n127 = Unbundle By Name(w428) -> ("Core.Close Panel on Exit?"=w427:bool)
        n128 = Select(t="UI: Front Panel State >> Close", s=w427, f="") -> (s? t:f=w423:string)
        n129 = call <vilib>:"Add State(s) to Queue__JKI_lib_State_Machine.vi"("State(s) in Front (\"\")"="UnRegister User Event" ("State(s) in Front (\"\")"), "State(s) in (\"\")"=w423, "State(s) at Back (\"\")"="Data: Save to INI\nData: Cleanup\nExit") -> ("States Out"=w426:string)  [unwired: 12 in]
        n130 = call <vilib>:"Add State(s) to Queue__JKI_lib_State_Machine.vi"("State(s) in Front (\"\")"=w426, "State(s) in (\"\")"=w431) -> ("States Out"=w430:string)  [unwired: 13 in]
      }
      frame "----- Action ------" {
      }
      frame "Action: Clear Non-exist JKISM" {
        n131 = Get Variant Attribute(Variant=w443) -> (duplicate Variant=w442:variant, names=w440:string[], values=w439:variant[])  [unwired: 3 in, 1 out]
        n132 = Variant To Data(type=T4[] [], Variant=w439) -> (data=w438:T4[])  [unwired: 1 in, 1 out]
        n133 = for {
          shift-right: [w459] -> w441
          shift-left: w442 -> [w460]
          tunnel: w440 -> [w458] mode=indexing
          tunnel: w438 -> [w457] mode=indexing
          n134 = Unbundle By Name(w457) -> ("Current State"=w455:string, "Name(\"\" to use uuid)"=w454:string)
          n135 = Search 1D Array(1D array=string[] ["<Remaining States>", "Exit"], element=w455) -> (index of element=w451:i32)  [unwired: 1 in]
          n136 = Match Pattern(string=w454, regular expression="^-") -> (offset past match=w452:i32)  [unwired: 1 in, 3 out]
          n137 = Greater Or Equal To 0?(x=w451) -> (x >= 0?=w449:bool)
          n138 = Greater Or Equal To 0?(x=w452) -> (x >= 0?=w450:bool)
          n139 = Or(x=w450, y=w449) -> (x .or. y?=w448:bool)
          n140 = case shown="True" w448 {
            tunnel: w460 -> [w461 w464]
            tunnel: [w461 w463] -> w459
            tunnel: w458 -> [_ w462]
            tunnel: w454 -> [_ _]
            tunnel: w455 -> [_ _]
            frame False {
            }
            frame True {
              n141 = Delete Variant Attribute(6:w462, 7:w464) -> (3:w463:variant)  [unwired: 1 in, 2 out]
            }
          }
        }
      }
    }
  }
